vi "KeyPad_Clear.vi"(0 "Display State In":T1, 9 "Container State":T2, 11 "error in (no error)":errorcluster) -> (4 "Display State Out":T1, 15 "error out":errorcluster)   [LabVIEW 2011, in "Keypad.xctl"]
uses:
  Keypad.xctl
  <vilib>/_xctls/Container State.ctl
  Keypad_State.ctl
  <vilib>/_xctls/XControlSupport.lvlib
panel:
  # "Add Controls & Indicators that form the parameters of the method here. Hook them to the connector pane. Do not delete the controls & indicators that are already hooked to the connector pane.\n \nTo setup the parameters  for this method, right click on this item in the Project Tree & select \"Configure Method...\"."
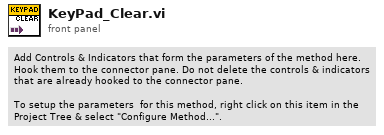
[diagram p1: front panel]
types:
  T1 = typedef "Keypad.xctl/Keypad_State.ctl" = cluster{"Numeric":dbl}
  T2 = typedef "XControlSupport.lvlib/Container State.ctl" = cluster{"Indicator?":bool, "Run Mode?":bool, " Refnum":refnum<vi>}
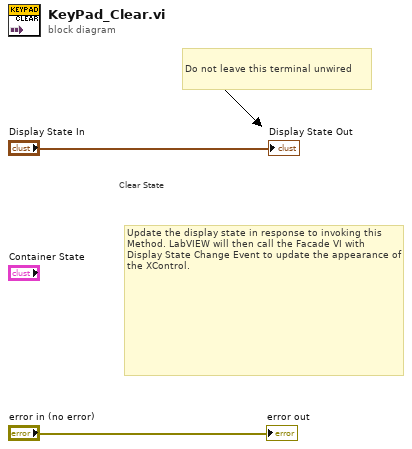
[diagram p0: block diagram]
diagram:
  # "Clear State"
  # "Do not leave this terminal unwired"
  # "Update the display state in response to invoking this Method. LabVIEW will then call the Facade VI with Display State Change Event to update the appearance of the XControl."
  "Display State Out" <- "Display State In"
  "error out" <- "error in (no error)"
